vi "To JSON String.vi"(8 "error in (no error)":errorcluster, 11 "error in":refnum<class "error.lvclass">) -> (0 "error out":errorcluster, 2 "JSON String":string, 3 "error out":refnum<class "error.lvclass">)   [LabVIEW 2016, in "error.lvclass"]
uses:
  error.lvclass
  <vilib>/NI/JSON Support for LabVIEW/JSON Data Classes/JSON Datatype/JSON Null.lvclass
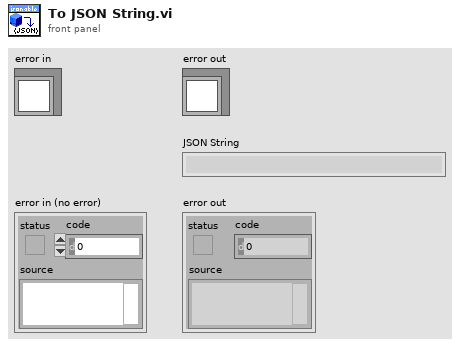
[diagram p1: front panel]
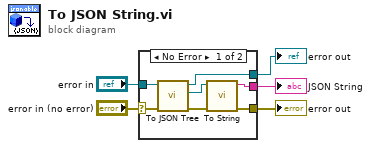
[diagram p0: block diagram]
diagram:
  n1 = case shown="No Error" "error in (no error)" {
    selector: "error in (no error)" -> [w11 w14]
    tunnel: [w7 w14] -> w4
    tunnel: [w10 w13] -> w2
    tunnel: "error in" -> [w12 w13]
    tunnel: [w8 _] -> w1
    frame No Error {
      n2 = call "To JSON Tree.vi"("error in (no error)"=w11, "error in"=w12) -> (0:"error out"=w6:errorcluster, "JSON out"=w9:refnum<class "JSON Null.lvclass">, 3:"error out"=w10:refnum<class "error.lvclass">)  [unwired: 7 in]
      n3 = call-dynamic "To String.vi"("error in (no error)"=w6, "JSON Datatype in"=w9) -> ("error out"=w7:errorcluster, "String"=w8:string)  [unwired: 8 in]
    }
    frame Error {
    }
  }
  "error out" <- w4
  "error out" <- w2
  "JSON String" <- w1
